vi "AD7609 config.vi"(5 "Device serial port":refnum<visa-resource-name>, 6 "Triggering mode":u8(ring) items=["Software", "Hardware"], 7 "N channels to read":u8(ring)=8 items=["1"=1, "2"=2, "3"=3, "4"=4, "5"=5, "6"=6, "7"=7, "8"=8], 8 "Input voltage range (V)":u8(ring)=1 items=["-5... +5 V", "-10... +10 V"], 9 "Oversampling ratio":u8(ring) items=["1", "2", "4", "8", "16", "32", "64"], 10 "Sampling rate (Hz)":sgl=1000.0, 11 "Number of samples":u32=1000) -> (0 "Config error out":errorcluster, 3 "Config read-back ok":bool=TRUE)   [LabVIEW 2015]
uses:
  <vilib>/Instr/_visa.llb/VISA Open Access Mode.ctl
  AD7609 global.vi
panel:
  out "Configuration read-back":string
  out "Configuration output":string
  # "30 kHz max. 8Ch\n54 kHz max. 1Ch"
  # "PN 25/11/2014, 17/08/2015 (removed timeout)"
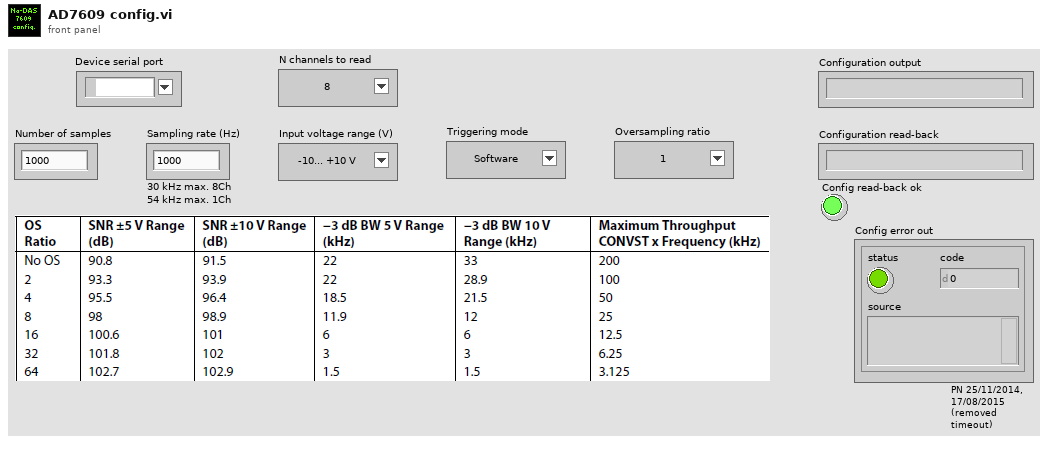
[diagram p1: front panel]
types:
  T1 = typedef "VISA Open Access Mode.ctl" = u32
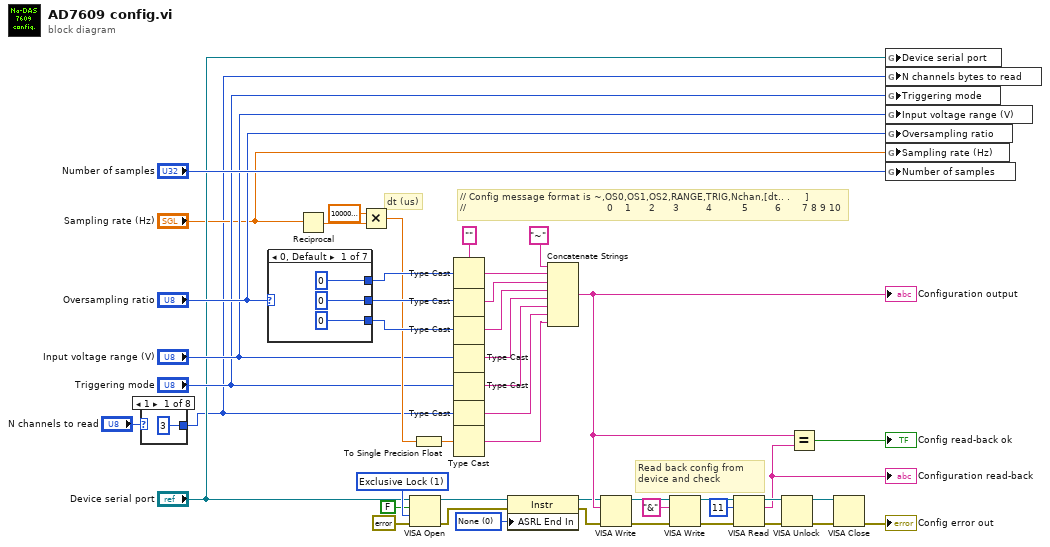
[diagram p0: block diagram]
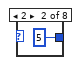
[diagram p2: hidden frame]
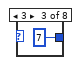
[diagram p3: hidden frame]
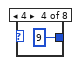
[diagram p4: hidden frame]
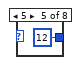
[diagram p5: hidden frame]
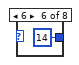
[diagram p6: hidden frame]
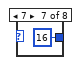
[diagram p7: hidden frame]
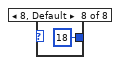
[diagram p8: hidden frame]
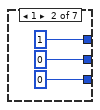
[diagram p9: hidden frame]
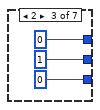
[diagram p10: hidden frame]
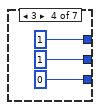
[diagram p11: hidden frame]
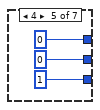
[diagram p12: hidden frame]
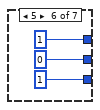
[diagram p13: hidden frame]
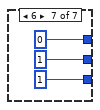
[diagram p14: hidden frame]
diagram:
  w5 = u16 0 items=["None", "Last Bit", "TermChar"] ("Serial Settings:End Mode for Reads")
  w34 = T1 1 items=["VISA Defaults"=0, "Exclusive Lock"=1, "Load Configured Settings"=4] ("Access Mode")
  w9 = ""
  # "Read back config from device and check"
  # "// Config message format is ~,OS0,OS1,OS2,RANGE,TRIG,Nchan,[dt.. .     ]\n//                                               0    1      2      3         4          5         6       7 8 9 10"
  # "dt (us)"
  n1 = case shown="1" "N channels to read" {
    tunnel: [u8 3 u8 5 u8 7 u8 9 u8 12 u8 14 u8 16 u8 18] -> w6
    frame 1 {
    }
    frame 2 {
    }
    frame 3 {
    }
    frame 4 {
    }
    frame 5 {
    }
    frame 6 {
    }
    frame 7 {
    }
    frame 8, Default {
    }
  }
  n2 = case shown="0, Default" "Oversampling ratio" {
    tunnel: [u8 0 u8 1 u8 0 u8 1 u8 0 u8 1 u8 0] -> w45
    tunnel: [u8 0 u8 0 u8 1 u8 1 u8 0 u8 0 u8 1] -> w44
    tunnel: [u8 0 u8 0 u8 0 u8 0 u8 1 u8 1 u8 1] -> w43
    frame 0, Default {
    }
    frame 1 {
    }
    frame 2 {
    }
    frame 3 {
    }
    frame 4 {
    }
    frame 5 {
    }
    frame 6 {
    }
  }
  n3 = Reciprocal(x="Sampling rate (Hz)") -> (1/x=w37:sgl)
  n4 = Multiply(x=sgl 1000000.0, y=w37) -> (x*y=w35:sgl)
  n5 = VISA Open(duplicate session (F)=FALSE, access mode=w34, error in (no error)=errorcluster {"status"=FALSE, "code"=0, "source"=""}, VISA resource name="Device serial port") -> (VISA resource name=w4:refnum<visa-resource-name>, error out=w1:errorcluster)  [unwired: 1 in]
  n6 = To Single Precision Float(number=w35) -> (single precision float=w22:sgl)
  n7 = Type Cast(type=w9, x=w45) -> (*(type *) &x=w42:string)
  n8 = Type Cast(type=w9, x=w44) -> (*(type *) &x=w41:string)
  n9 = Type Cast(type=w9, x=w43) -> (*(type *) &x=w40:string)
  n10 = Type Cast(type=w9, x="Input voltage range (V)") -> (*(type *) &x=w39:string)
  n11 = Type Cast(type=w9, x="Triggering mode") -> (*(type *) &x=w38:string)
  n12 = Type Cast(type=w9, x=w6) -> (*(type *) &x=w8:string)
  n13 = Type Cast(type=w9, x=w22) -> (*(type *) &x=w10:string)
  n14 = property class="Instr"(reference=w4, error in=w1, "ASRL End In"=w5) -> (reference out=w3:refnum<visa-resource-name>, error out=w2:errorcluster)
  n15 = Concatenate Strings("~", w42, w41, w40, w39, w38, w8, w10) -> (w12:string)
  "Configuration output" <- w12
  n16 = VISA Write(VISA resource name=w3, write buffer=w12, error in (no error)=w2) -> (VISA resource name out=w20:refnum<visa-resource-name>, error out=w21:errorcluster)  [unwired: 1 out]
  n17 = VISA Write(VISA resource name=w20, write buffer="&", error in (no error)=w21) -> (VISA resource name out=w18:refnum<visa-resource-name>, error out=w17:errorcluster)  [unwired: 1 out]
  n18 = VISA Read(VISA resource name=w18, byte count=u32 11, error in (no error)=w17) -> (VISA resource name out=w15:refnum<visa-resource-name>, read buffer=w13:string, error out=w16:errorcluster)  [unwired: 1 out]
  "Configuration read-back" <- w13
  n19 = VISA Unlock(8:w16, 11:w15) -> (0:w31:errorcluster, 3:w32:refnum<visa-resource-name>)
  n20 = Equal?(x=w12, y=w13) -> (x = y?=→"Config read-back ok":bool)
  n21 = VISA Close(VISA resource name=w32, error in (no error)=w31) -> (error out=→"Config error out":errorcluster)
  n22 = global write "AD7609 global.vi" "Device serial port"("Device serial port") -> ()
  n23 = global write "AD7609 global.vi" "N channels bytes to read"(w6) -> ()
  n24 = global write "AD7609 global.vi" "Triggering mode"("Triggering mode") -> ()
  n25 = global write "AD7609 global.vi" "Input voltage range (V)"("Input voltage range (V)") -> ()
  n26 = global write "AD7609 global.vi" "Oversampling ratio"("Oversampling ratio") -> ()
  n27 = global write "AD7609 global.vi" "Sampling rate (Hz)"("Sampling rate (Hz)") -> ()
  n28 = global write "AD7609 global.vi" "Number of samples"("Number of samples") -> ()
